vi "BlackBox Configurator.vi"() -> ()   [LabVIEW 2015]
doc: "Example VI that demonstrates all library features."
uses:
  PL BlackBox Modbus Client.lvclass
panel:
  in  "read device info":bool=TRUE
  in  "read configuration":bool=TRUE
  out "hardware interface state":T1
  in  "server configuration":T2 {"protocol" items=["RTU", "ASCII", "TCP"]}
  out "server type":u16(ring) items=["Unknown", "UART server", "Network server", "Modbus serial server", "Modbus TCP server"]
  out "hardware interface type":u16(ring) items=["Unknown", "UART", "Network interface", "Ethernet", "Wi-Fi"]
  in  "hardware interface configuration":T3 {"flow control" items=["none", "rts", "cts", "rts/cts"]; "stop bits" items=["1", "1.5", "2"]; "parity" items=["none", "even", "odd"]}
  out "server types":u16[](array[numeric])
  in  "server":u16(ring)
  out "hardware interface types":u16[](array[numeric])
  in  "hardware interface":u16(ring)
  in  "save configuration":bool
  out "uid":string
  out "firmware":string
  out "hardware":string
  in  "restart":bool
  in  "clear restarted flag":bool
  in  "device name":string
  out "PLBB":refnum<class "PL BlackBox Modbus Client.lvclass">
  in  "interface":enum32{"serial", "TCP"}(tab)
  in  "serial settings":T4={"port"="", "protocol"=enum."RTU", "address"=1, "baud rate"=115200, "data bits"=8, "parity"=2, "stop bits"=10, "flow control"=0} {"flow control" items=["None", "XON/XOFF", "RTS/CTS", "XON/XOFF & RTS/CTS", "DTR/DSR", "XON/XOFF & DTR/DSR"]; "stop bits" items=["1.0"=10, "1.5"=15, "2.0"=20]; "parity" items=["None", "Odd", "Even", "Mark", "Space"]}
  in  "TCP settings":T5={"ip address"="192.168.1.1", "port"=502, "station address"=255}
  out "error":errorcluster
  in  "stop":bool
  out "restarted":bool
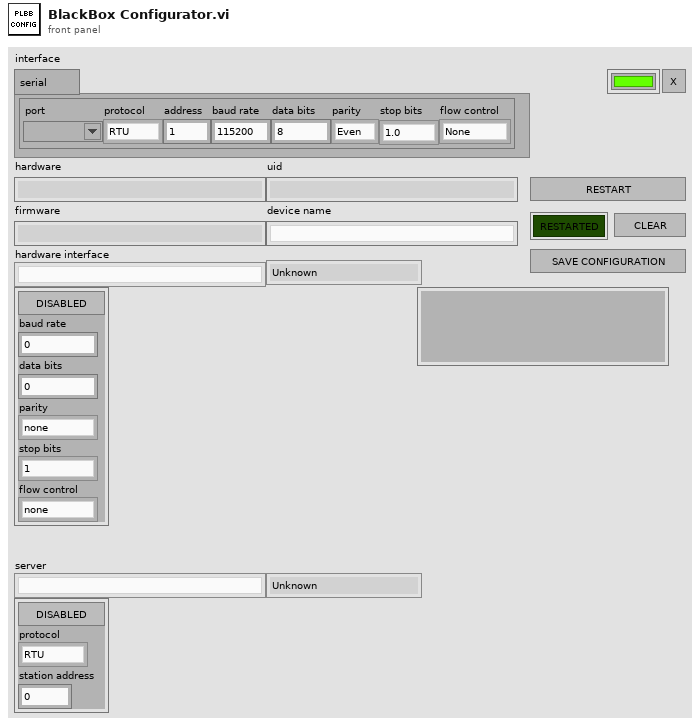
[diagram p1: front panel]
types:
  T1 = cluster{"connected":bool, "IPv6":cluster{"link-local address":string}}
  T2 = cluster{"enabled":bool, "port":u16, "max number of clients":u16, "protocol":u16, "station address":u16}
  T3 = cluster{"enabled":bool, "baud rate":u32, "data bits":u16, "parity":u16, "stop bits":u16, "flow control":u16, "IPv4":cluster{"DHCP client enabled":bool, "address":string, "netmask":string, "gateway":string}, "IPv6":cluster{"DHCP client enabled":bool, "global address":string}, "SSID":string, "password":string}
  T4 = cluster{"port":refnum<visa-resource-name>, "protocol":enum16{"RTU", "ASCII"}, "address":u8, "baud rate":u32, "data bits":u16, "parity":u16, "stop bits":u16, "flow control":u16}
  T5 = cluster{"ip address":string, "port":u16, "station address":u8}
  T6 = cluster{"connected":bool, "network interface":cluster{"IPv6":cluster{"link-local address":string}}}
  T7 = cluster{"enabled":bool, "UART":cluster{"baud rate":u32, "data bits":u16, "parity":u16, "stop bits":u16, "flow control":u16}, "network interface":cluster{"IPv4":cluster{"DHCP client enabled":bool, "address":string, "netmask":string, "gateway":string}, "IPv6":cluster{"DHCP client enabled":bool, "global address":string}, "Wi-Fi":cluster{"SSID":string, "password":string}}}
  T8 = cluster{"hardware":cluster{"name":string, "version":cluster{"major":u16, "minor":u16, "patch":u16}, "uid":string}, "firmware":cluster{"name":string, "version":cluster{"major":u16, "minor":u16, "patch":u16}}, "number of hardware interfaces":u16, "number of servers":u16}
  T9 = cluster{"DHCP client enabled":bool, "address":string, "netmask":string, "gateway":string}
  T10 = cluster{"DHCP client enabled":bool, "global address":string}
  T11 = cluster{"enabled":bool, "network server":cluster{"port":u16, "max number of clients":u16}, "Modbus server":cluster{"protocol":u16, "station address":u16}}
  T12 = cluster{"enabled":bool, "baud rate":u32, "data bits":u16, "parity":u16, "stop bits":u16, "flow control":u16}
  T13 = cluster{"enabled":bool, "IPv4":cluster{"DHCP client enabled":bool, "address":string, "netmask":string, "gateway":string}, "IPv6":cluster{"DHCP client enabled":bool, "global address":string}}
  T14 = cluster{"enabled":bool, "IPv4":cluster{"DHCP client enabled":bool, "address":string, "netmask":string, "gateway":string}, "IPv6":cluster{"DHCP client enabled":bool, "global address":string}, "SSID":string, "password":string}
  T15 = cluster{"enabled":bool, "port":u16, "max number of clients":u16}
  T16 = cluster{"enabled":bool, "protocol":u16, "station address":u16}
  T17 = cluster{"enabled":bool, "protocol":u16, "station address":u16, "port":u16, "max number of clients":u16}
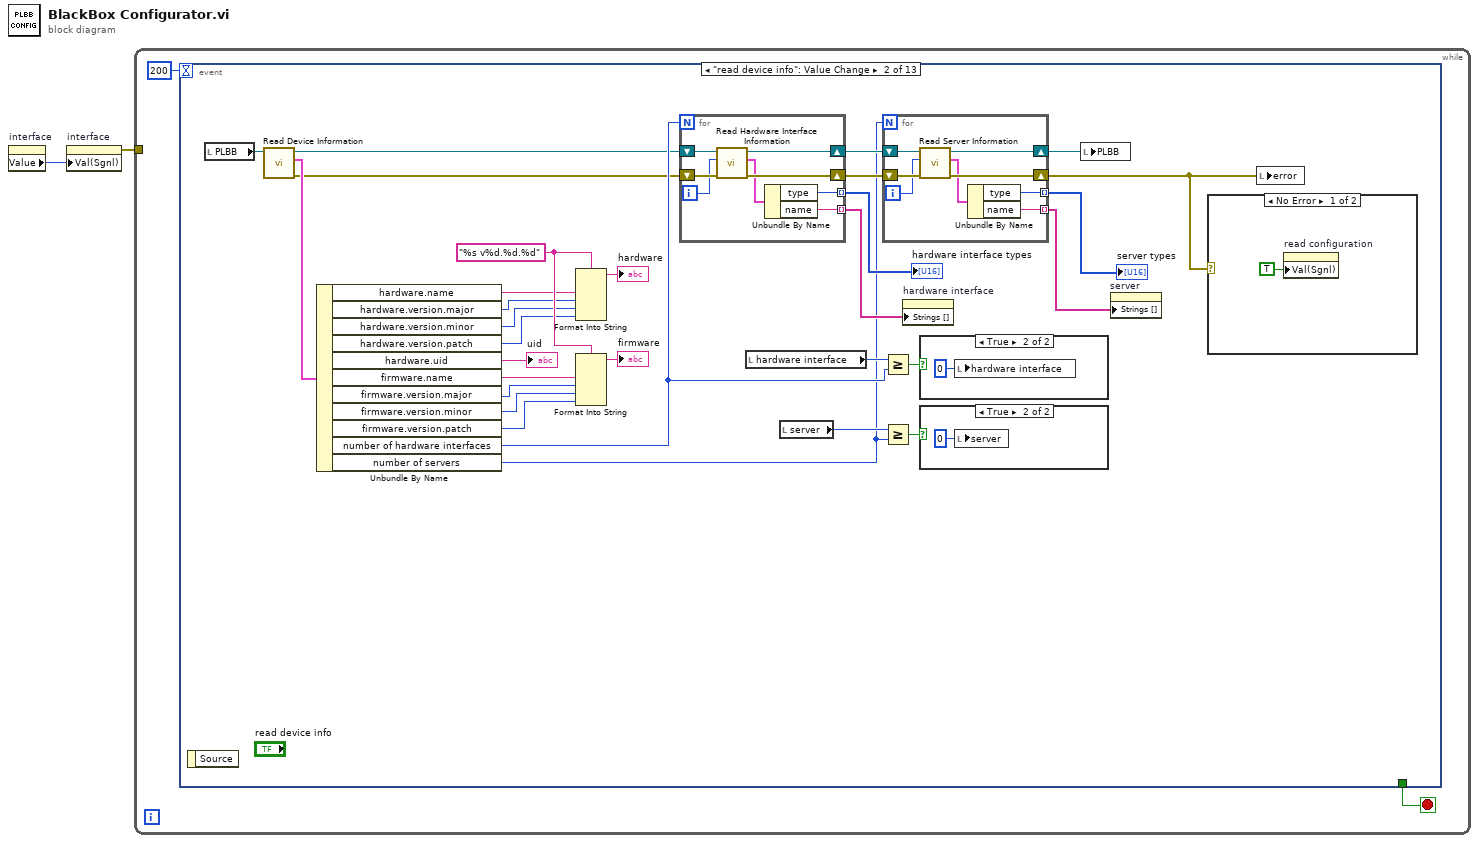
[diagram p0: block diagram]
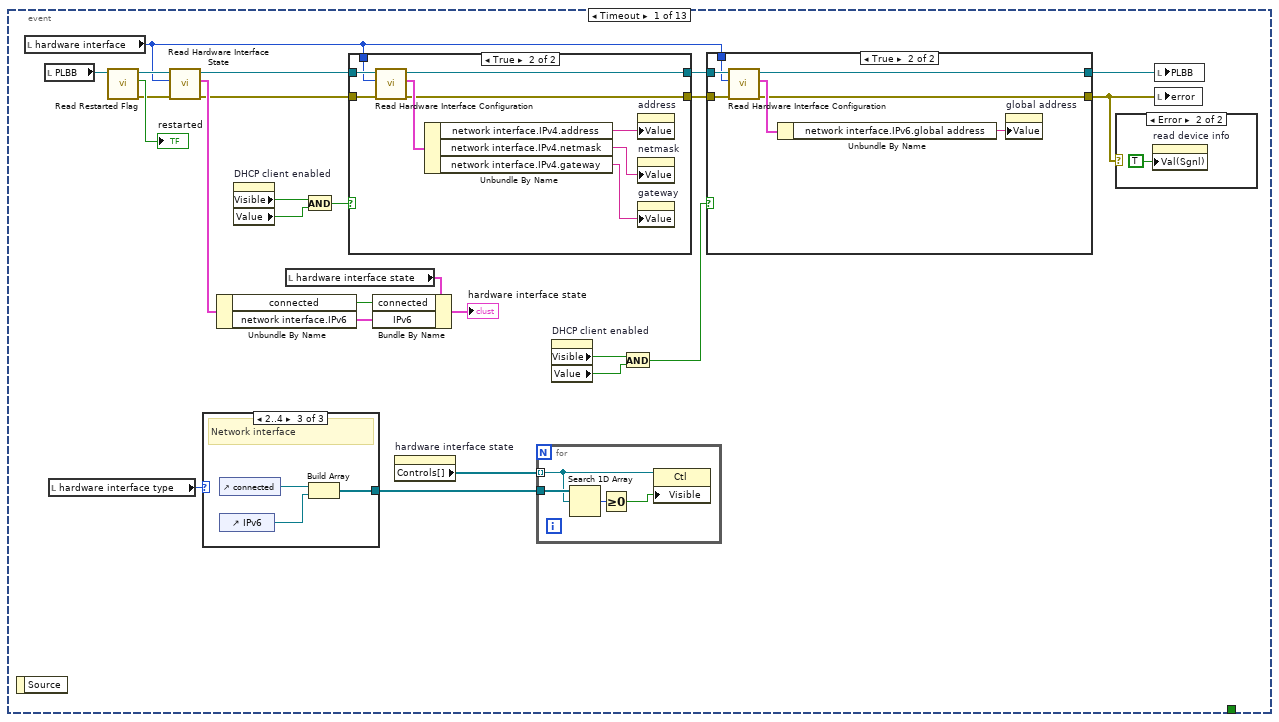
[diagram p2: hidden frame]
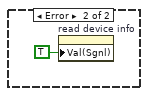
[diagram p8: hidden frame]
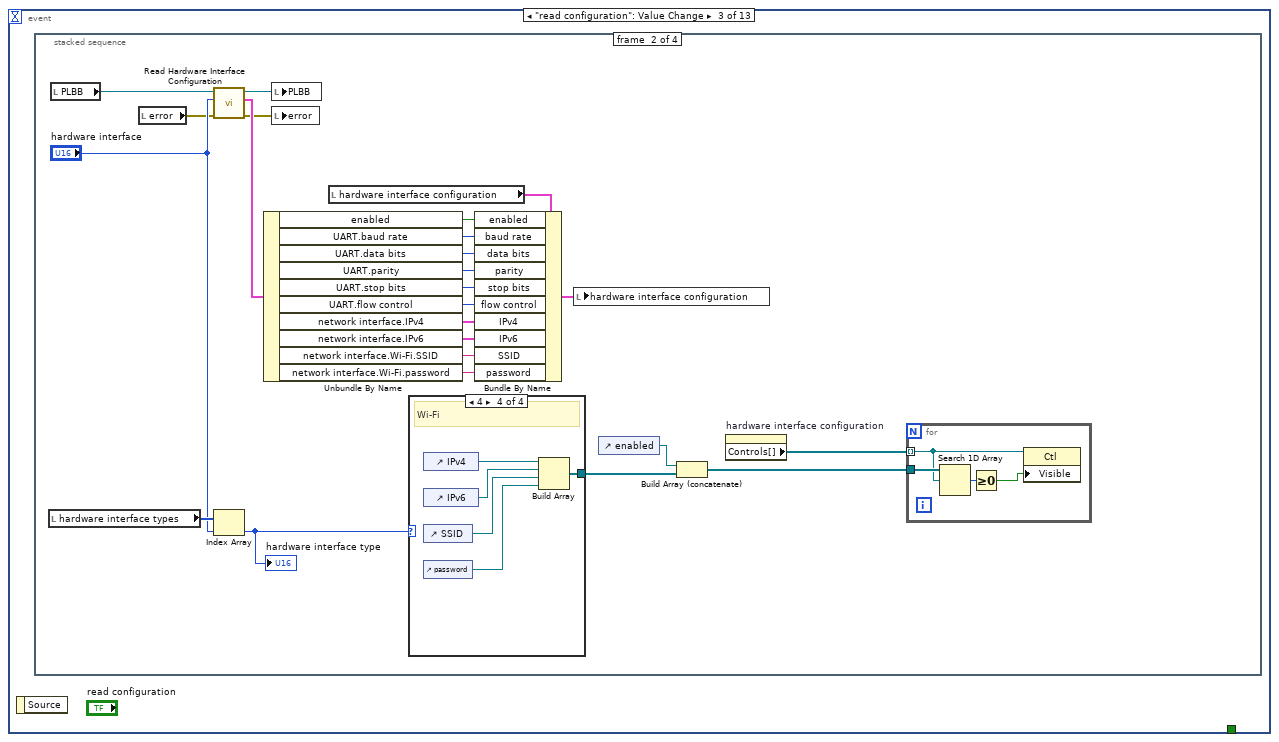
[diagram p11: hidden frame]
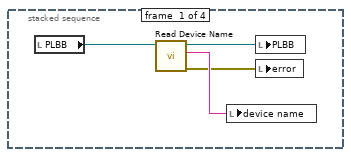
[diagram p12: hidden frame]
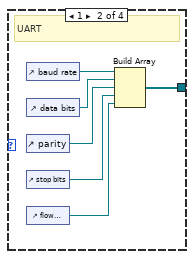
[diagram p14: hidden frame]
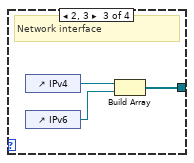
[diagram p15: hidden frame]
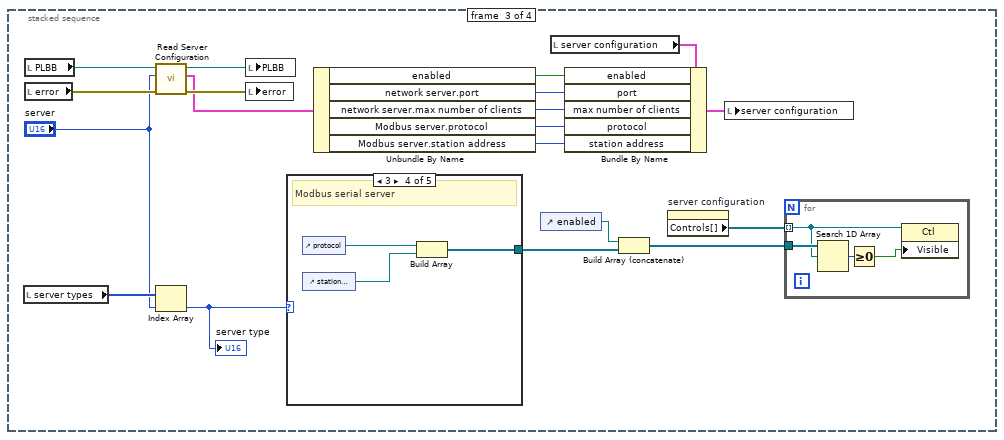
[diagram p16: hidden frame]
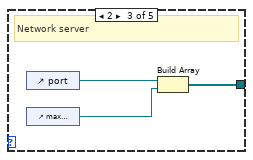
[diagram p19: hidden frame]
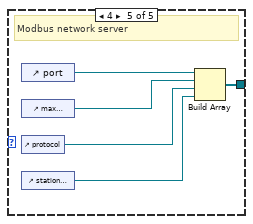
[diagram p20: hidden frame]
diagram:
  n1 = property on="interface" class="TabCtl (strict)"() -> ("Value"=w2:enum32{"serial", "TCP"})  [unwired: 2 in, 2 out]
  n2 = property on="interface" class="TabCtl (strict)"("Val(Sgnl)"=w2) -> (error out=w1:errorcluster)  [unwired: 2 in, 1 out]
  n3 = while {
    tunnel: w1 -> [_]
    stop <- w3 stop-if-true
    n4 = event shown="[1] \"read device info\": Value Change" {
      selector: _ -> [_ _ _ _ _ _ _ _ _ _ _ _ _]
      dyn-events: _ -> [_ _ _ _ _ _ _ _ _ _ _ _ _]
      timeout: 200 -> [_ _ _ _ _ _ _ _ _ _ _ _ _]
      tunnel: [_ _ _ _ _ _ _ _ _ _ _ _ TRUE ("stop")] -> w3
      event Timeout {
        n5 = event-data() -> ()  [unwired: 1 in, 1 out]
        n6 = local read "hardware interface"() -> (w13:u16)
        n7 = local read "PLBB"() -> (w24:refnum<class "PL BlackBox Modbus Client.lvclass">)
        n8 = local read "hardware interface type"() -> (w7:u16)
        n9 = call "Read Restarted Flag.vi"("PLBB in"=w24) -> ("error out"=w21:errorcluster, "restarted flag"=→"restarted":bool, "PLBB out"=w22:refnum<class "PL BlackBox Modbus Client.lvclass">)  [unwired: 8 in]
        n10 = call "Read Hardware Interface State.vi"("error in (no error)"=w21, "hardware interface index"=w13, "PLBB in"=w22) -> ("error out"=w16:errorcluster, "hardware interface state"=w28:T6, "PLBB out"=w18:refnum<class "PL BlackBox Modbus Client.lvclass">)  [unwired: 6 in]
        n11 = case shown="2..4" w7 {
          tunnel: [_ _ w36] -> w5
          frame 0, Default {
          }
          frame 1 {
            # "UART"
          }
          frame 2..4 {
            # "Network interface"
            n12 = control-ref of="connected"() -> (w34:refnum<vi>)
            n13 = control-ref of="IPv6"() -> (w35:refnum<vi>)
            n14 = Build Array(w34, w35) -> (w36:refnum<vi>[])
          }
        }
        n15 = Unbundle By Name(w28) -> ("connected"=w26:bool, "network interface.IPv6"=w25:cluster{"link-local address":string})
        n16 = property on="DHCP client enabled" class="Bool (strict)"() -> ("Visible"=w20:bool, "Value"=w19:bool)  [unwired: 2 in, 2 out]
        n17 = local read "hardware interface state"() -> (w27:T1)
        n18 = And(x=w20, y=w19) -> (x .and. y?=w17:bool)
        n19 = case shown="True" w17 {
          tunnel: w18 -> [w48 w57]
          tunnel: w16 -> [w47 w56]
          tunnel: w13 -> [_ w55]
          tunnel: [w47 w50] -> w11
          tunnel: [w48 w49] -> w12
          frame False {
          }
          frame True {
            n20 = call "Read Hardware Interface Configuration.vi"("error in (no error)"=w56, "hardware interface index"=w55, "PLBB in"=w57) -> ("error out"=w50:errorcluster, "hardware interface configuration"=w54:T7, "PLBB out"=w49:refnum<class "PL BlackBox Modbus Client.lvclass">)  [unwired: 6 in]
            n21 = Unbundle By Name(w54) -> ("network interface.IPv4.address"=w53:string, "network interface.IPv4.netmask"=w52:string, "network interface.IPv4.gateway"=w51:string)
            n22 = property on="address" class="Str"("Value"=w53) -> ()  [unwired: 2 in, 2 out]
            n23 = property on="netmask" class="Str"("Value"=w52) -> ()  [unwired: 2 in, 2 out]
            n24 = property on="gateway" class="Str"("Value"=w51) -> ()  [unwired: 2 in, 2 out]
          }
        }
        n25 = Bundle By Name(cluster=w27, "connected"=w26, "IPv6"=w25) -> (→"hardware interface state":T1)
        n26 = property on="hardware interface state" class="Clust (strict)"() -> ("Controls[]"=w6:refnum<vi>[])  [unwired: 2 in, 2 out]
        n27 = for {
          tunnel: w6 -> [w32] mode=indexing
          tunnel: w5 -> [w33]
          n28 = Search 1D Array(1D array=w33, element=w32) -> (index of element=w31:i32)  [unwired: 1 in]
          n29 = Greater Or Equal To 0?(x=w31) -> (x >= 0?=w30:bool)
          n30 = property class="Ctl"(reference=w32, "Visible"=w30) -> ()  [unwired: 1 in, 2 out]
        }
        n31 = property on="DHCP client enabled" class="Bool (strict)"() -> ("Visible"=w14:bool, "Value"=w15:bool)  [unwired: 2 in, 2 out]
        n32 = And(x=w14, y=w15) -> (x .and. y?=w9:bool)
        n33 = case shown="True" w9 {
          tunnel: w12 -> [w39 w46]
          tunnel: w11 -> [w38 w45]
          tunnel: w13 -> [_ w44]
          tunnel: [w38 w41] -> w8
          tunnel: [w39 w40] -> w10
          frame False {
          }
          frame True {
            n34 = call "Read Hardware Interface Configuration.vi"("error in (no error)"=w45, "hardware interface index"=w44, "PLBB in"=w46) -> ("error out"=w41:errorcluster, "hardware interface configuration"=w43:T7, "PLBB out"=w40:refnum<class "PL BlackBox Modbus Client.lvclass">)  [unwired: 6 in]
            n35 = Unbundle By Name(w43) -> ("network interface.IPv6.global address"=w42:string)
            n36 = property on="global address" class="Str"("Value"=w42) -> ()  [unwired: 2 in, 2 out]
          }
        }
        n37 = case shown="Error" w8 {
          frame No Error {
          }
          frame Error {
            n38 = property on="read device info" class="Bool (strict)"("Val(Sgnl)"=TRUE ("Value (Signaling)")) -> ()  [unwired: 2 in, 2 out]
          }
        }
        n39 = local write "PLBB"(w10) -> ()
        n40 = local write "error"(w8) -> ()
      }
      event "read device info": Value Change {
        w85 = "%s v%d.%d.%d" ("format string")
        n41 = event-data() -> ()  [unwired: 1 in, 1 out]
        n42 = local read "PLBB"() -> (w87:refnum<class "PL BlackBox Modbus Client.lvclass">)
        n43 = call "Read Device Information.vi"("PLBB in"=w87) -> ("error out"=w58:errorcluster, "device information"=w86:T8, "PLBB out"=w59:refnum<class "PL BlackBox Modbus Client.lvclass">)  [unwired: 8 in]
        n44 = Unbundle By Name(w86) -> ("hardware.name"=w84:string, "hardware.version.major"=w83:u16, "hardware.version.minor"=w82:u16, "hardware.version.patch"=w81:u16, "hardware.uid"=→"uid":string, "firmware.name"=w80:string, "firmware.version.major"=w79:u16, "firmware.version.minor"=w78:u16, "firmware.version.patch"=w77:u16, "number of hardware interfaces"=w64:u16, "number of servers"=w61:u16)
        n45 = Format Into String(format string=w85, w84, w83, w82, w81) -> (resulting string=→"hardware":string)  [unwired: 2 in, 1 out]
        n46 = Format Into String(format string=w85, w80, w79, w78, w77) -> (resulting string=→"firmware":string)  [unwired: 2 in, 1 out]
        n47 = for {
          N: w64 -> [_]
          shift-right: [w104] -> w69
          shift-left: w59 -> [w107]
          shift-right: [w105] -> w68
          shift-left: w58 -> [w106]
          tunnel: [w101] -> w73 mode=indexing
          tunnel: [w100] -> w72 mode=indexing
          i -> [w103]
          n48 = call "Read Hardware Interface Information.vi"("error in (no error)"=w106, "hardware interface index"=w103, "PLBB in"=w107) -> ("error out"=w105:errorcluster, "hardware interface information"=w102:cluster{"type":u16, "name":string}, "PLBB out"=w104:refnum<class "PL BlackBox Modbus Client.lvclass">)  [unwired: 6 in]
          n49 = Unbundle By Name(w102) -> ("type"=w101:u16, "name"=w100:string)
        }
        "hardware interface types" <- w73
        n50 = local read "hardware interface"() -> (w65:u16)
        n51 = local read "server"() -> (w63:u16)
        n52 = for {
          N: w61 -> [_]
          shift-right: [w96] -> w70
          shift-left: w69 -> [w99]
          shift-right: [w97] -> w60
          shift-left: w68 -> [w98]
          tunnel: [w93] -> w71 mode=indexing
          tunnel: [w92] -> w67 mode=indexing
          i -> [w95]
          n53 = call "Read Server Information.vi"("error in (no error)"=w98, "server index"=w95, "PLBB in"=w99) -> ("error out"=w97:errorcluster, "server information"=w94:cluster{"type":u16, "name":string}, "PLBB out"=w96:refnum<class "PL BlackBox Modbus Client.lvclass">)  [unwired: 6 in]
          n54 = Unbundle By Name(w94) -> ("type"=w93:u16, "name"=w92:string)
        }
        "server types" <- w71
        n55 = Greater Or Equal?(x=w65, y=w64) -> (x >= y?=w66:bool)
        n56 = Greater Or Equal?(x=w63, y=w61) -> (x >= y?=w62:bool)
        n57 = property on="hardware interface" class="Ring (strict)"("Strings []"=w72) -> ()  [unwired: 2 in, 2 out]
        n58 = case shown="True" w66 {
          frame False {
          }
          frame True {
            n59 = local write "hardware interface"(u16 0) -> ()
          }
        }
        n60 = case shown="True" w62 {
          frame False {
          }
          frame True {
            n61 = local write "server"(u16 0) -> ()
          }
        }
        n62 = local write "PLBB"(w70) -> ()
        n63 = property on="server" class="Ring (strict)"("Strings []"=w67) -> ()  [unwired: 2 in, 2 out]
        n64 = case shown="No Error" w60 {
          frame No Error {
            n65 = property on="read configuration" class="Bool (strict)"("Val(Sgnl)"=TRUE ("Value (Signaling)")) -> ()  [unwired: 2 in, 2 out]
          }
          frame Error {
            n66 = property on="read device info" class="Bool (strict)"("Val(Sgnl)"=TRUE ("Value (Signaling)")) -> ()  [unwired: 2 in, 2 out]
          }
        }
        n67 = local write "error"(w60) -> ()
      }
      event "read configuration": Value Change {
        n68 = event-data() -> ()  [unwired: 1 in, 1 out]
        n69 = stacked-sequence {
          frame #0 {
            n70 = local read "PLBB"() -> (w110:refnum<class "PL BlackBox Modbus Client.lvclass">)
            n71 = call "Read Device Name.vi"("PLBB in"=w110) -> ("error out"=w108:errorcluster, "device name"=w111:string, "PLBB out"=w109:refnum<class "PL BlackBox Modbus Client.lvclass">)  [unwired: 8 in]
            n72 = local write "device name"(w111) -> ()
            n73 = local write "PLBB"(w109) -> ()
            n74 = local write "error"(w108) -> ()
          }
          frame #1 {
            n75 = local read "hardware interface types"() -> (w134:u16[])
            n76 = local read "PLBB"() -> (w135:refnum<class "PL BlackBox Modbus Client.lvclass">)
            n77 = local read "error"() -> (w112:errorcluster)
            n78 = call "Read Hardware Interface Configuration.vi"("error in (no error)"=w112, "hardware interface index"="hardware interface", "PLBB in"=w135) -> ("error out"=w113:errorcluster, "hardware interface configuration"=w133:T7, "PLBB out"=w114:refnum<class "PL BlackBox Modbus Client.lvclass">)  [unwired: 6 in]
            n79 = Index Array(array=w134, index="hardware interface") -> (element=w122:u16)
            "hardware interface type" <- w122
            n80 = Unbundle By Name(w133) -> ("enabled"=w131:bool, "UART.baud rate"=w130:u32, "UART.data bits"=w129:u16, "UART.parity"=w128:u16, "UART.stop bits"=w127:u16, "UART.flow control"=w126:u16, "network interface.IPv4"=w125:T9, "network interface.IPv6"=w124:T10, "network interface.Wi-Fi.SSID"=w115:string, "network interface.Wi-Fi.password"=w116:string)
            n81 = local write "PLBB"(w114) -> ()
            n82 = local write "error"(w113) -> ()
            n83 = local read "hardware interface configuration"() -> (w132:T3)
            n84 = case shown="4" w122 {
              tunnel: [_ w140 w146 w149] -> w121
              frame 0, Default {
              }
              frame 1 {
                # "UART"
                n85 = control-ref of="baud rate"() -> (w141:refnum<vi>)
                n86 = control-ref of="data bits"() -> (w142:refnum<vi>)
                n87 = control-ref of="parity"() -> (w143:refnum<vi>)
                n88 = control-ref of="stop bits"() -> (w144:refnum<vi>)
                n89 = control-ref of="flow control"() -> (w145:refnum<vi>)
                n90 = Build Array(w141, w142, w143, w144, w145) -> (w140:refnum<vi>[])
              }
              frame 2, 3 {
                # "Network interface"
                n91 = control-ref of="IPv4"() -> (w147:refnum<vi>)
                n92 = control-ref of="IPv6"() -> (w148:refnum<vi>)
                n93 = Build Array(w147, w148) -> (w146:refnum<vi>[])
              }
              frame 4 {
                # "Wi-Fi"
                n94 = control-ref of="IPv4"() -> (w150:refnum<vi>)
                n95 = control-ref of="IPv6"() -> (w151:refnum<vi>)
                n96 = control-ref of="SSID"() -> (w152:refnum<vi>)
                n97 = control-ref of="password"() -> (w153:refnum<vi>)
                n98 = Build Array(w150, w151, w152, w153) -> (w149:refnum<vi>[])
              }
            }
            n99 = Bundle By Name(cluster=w132, "enabled"=w131, "baud rate"=w130, "data bits"=w129, "parity"=w128, "stop bits"=w127, "flow control"=w126, "IPv4"=w125, "IPv6"=w124, "SSID"=w115, "password"=w116) -> (w123:T3)
            n100 = local write "hardware interface configuration"(w123) -> ()
            n101 = control-ref of="enabled"() -> (w120:refnum<vi>)
            n102 = Build Array (concatenate)(w120, w121) -> (w118:refnum<vi>[])
            n103 = property on="hardware interface configuration" class="Clust (strict)"() -> ("Controls[]"=w119:refnum<vi>[])  [unwired: 2 in, 2 out]
            n104 = for {
              tunnel: w119 -> [w138] mode=indexing
              tunnel: w118 -> [w139]
              n105 = Search 1D Array(1D array=w139, element=w138) -> (index of element=w137:i32)  [unwired: 1 in]
              n106 = Greater Or Equal To 0?(x=w137) -> (x >= 0?=w136:bool)
              n107 = property class="Ctl"(reference=w138, "Visible"=w136) -> ()  [unwired: 1 in, 2 out]
            }
          }
          frame #2 {
            n108 = local read "server types"() -> (w168:u16[])
            n109 = local read "PLBB"() -> (w172:refnum<class "PL BlackBox Modbus Client.lvclass">)
            n110 = local read "error"() -> (w171:errorcluster)
            n111 = call "Read Server Configuration.vi"("error in (no error)"=w171, "server index"="server", "PLBB in"=w172) -> ("error out"=w169:errorcluster, "server configuration"=w167:T11, "PLBB out"=w170:refnum<class "PL BlackBox Modbus Client.lvclass">)  [unwired: 6 in]
            n112 = Index Array(array=w168, index="server") -> (element=w154:u16)
            "server type" <- w154
            n113 = local write "PLBB"(w170) -> ()
            n114 = local write "error"(w169) -> ()
            n115 = case shown="3" w154 {
              tunnel: [_ _ w177 w180 w183] -> w159
              frame 0, Default {
              }
              frame 1 {
                # "UART server"
              }
              frame 2 {
                # "Network server"
                n116 = control-ref of="port"() -> (w178:refnum<vi>)
                n117 = control-ref of="max number of clients"() -> (w179:refnum<vi>)
                n118 = Build Array(w178, w179) -> (w177:refnum<vi>[])
              }
              frame 3 {
                # "Modbus serial server"
                n119 = control-ref of="protocol"() -> (w181:refnum<vi>)
                n120 = control-ref of="station address"() -> (w182:refnum<vi>)
                n121 = Build Array(w181, w182) -> (w180:refnum<vi>[])
              }
              frame 4 {
                # "Modbus network server"
                n122 = control-ref of="port"() -> (w184:refnum<vi>)
                n123 = control-ref of="max number of clients"() -> (w185:refnum<vi>)
                n124 = control-ref of="protocol"() -> (w186:refnum<vi>)
                n125 = control-ref of="station address"() -> (w187:refnum<vi>)
                n126 = Build Array(w184, w185, w186, w187) -> (w183:refnum<vi>[])
              }
            }
            n127 = Unbundle By Name(w167) -> ("enabled"=w165:bool, "network server.port"=w164:u16, "network server.max number of clients"=w163:u16, "Modbus server.protocol"=w162:u16, "Modbus server.station address"=w161:u16)
            n128 = control-ref of="enabled"() -> (w158:refnum<vi>)
            n129 = local read "server configuration"() -> (w166:T2)
            n130 = Bundle By Name(cluster=w166, "enabled"=w165, "port"=w164, "max number of clients"=w163, "protocol"=w162, "station address"=w161) -> (w160:T2)
            n131 = Build Array (concatenate)(w158, w159) -> (w156:refnum<vi>[])
            n132 = property on="server configuration" class="Clust (strict)"() -> ("Controls[]"=w157:refnum<vi>[])  [unwired: 2 in, 2 out]
            n133 = local write "server configuration"(w160) -> ()
            n134 = for {
              tunnel: w157 -> [w175] mode=indexing
              tunnel: w156 -> [w176]
              n135 = Search 1D Array(1D array=w176, element=w175) -> (index of element=w174:i32)  [unwired: 1 in]
              n136 = Greater Or Equal To 0?(x=w174) -> (x >= 0?=w173:bool)
              n137 = property class="Ctl"(reference=w175, "Visible"=w173) -> ()  [unwired: 1 in, 2 out]
            }
          }
          frame #3 {
            n138 = local read "error"() -> (w188:errorcluster)
            n139 = case shown="Error" w188 {
              frame No Error {
              }
              frame Error {
                n140 = property on="read device info" class="Bool (strict)"("Val(Sgnl)"=TRUE ("Value (Signaling)")) -> ()  [unwired: 2 in, 2 out]
              }
            }
          }
        }
      }
      event "restart": Value Change {
        n141 = event-data() -> ()  [unwired: 1 in, 1 out]
        n142 = local read "PLBB"() -> (w190:refnum<class "PL BlackBox Modbus Client.lvclass">)
        n143 = call "Restart.vi"("PLBB in"=w190) -> ("error out"=w192:errorcluster, "PLBB out"=w191:refnum<class "PL BlackBox Modbus Client.lvclass">)  [unwired: 9 in]
        n144 = local write "PLBB"(w191) -> ()
        n145 = local write "error"(w192) -> ()
      }
      event "clear restarted flag": Value Change {
        n146 = event-data() -> ()  [unwired: 1 in, 1 out]
        n147 = local read "PLBB"() -> (w193:refnum<class "PL BlackBox Modbus Client.lvclass">)
        n148 = call "Clear Restarted Flag.vi"("PLBB in"=w193) -> ("error out"=w195:errorcluster, "PLBB out"=w194:refnum<class "PL BlackBox Modbus Client.lvclass">)  [unwired: 9 in]
        n149 = local write "PLBB"(w194) -> ()
        n150 = local write "error"(w195) -> ()
      }
      event "save configuration": Value Change {
        n151 = event-data() -> ()  [unwired: 1 in, 1 out]
        n152 = local read "PLBB"() -> (w196:refnum<class "PL BlackBox Modbus Client.lvclass">)
        n153 = call "Save Configuration.vi"("PLBB in"=w196) -> ("error out"=w198:errorcluster, "PLBB out"=w197:refnum<class "PL BlackBox Modbus Client.lvclass">)  [unwired: 9 in]
        n154 = local write "PLBB"(w197) -> ()
        n155 = local write "error"(w198) -> ()
      }
      event "device name": Value Change {
        n156 = event-data() -> ()  [unwired: 1 in, 1 out]
        n157 = local read "PLBB"() -> (w201:refnum<class "PL BlackBox Modbus Client.lvclass">)
        n158 = call "Write Device Name.vi"("device name"="device name", "PLBB in"=w201) -> ("error out"=w203:errorcluster, "PLBB out"=w202:refnum<class "PL BlackBox Modbus Client.lvclass">)  [unwired: 8 in]
        n159 = local write "PLBB"(w202) -> ()
        n160 = local write "error"(w203) -> ()
        n161 = property on="read configuration" class="Bool (strict)"("Val(Sgnl)"=TRUE ("Value (Signaling)")) -> ()  [unwired: 2 in, 2 out]
      }
      event "hardware interface", "server": Value Change {
        n162 = event-data() -> ()  [unwired: 1 in, 6 out]
        n163 = property on="read configuration" class="Bool (strict)"("Val(Sgnl)"=TRUE ("Value (Signaling)")) -> ()  [unwired: 2 in, 2 out]
      }
      event "hardware interface configuration": Value Change {
        n164 = event-data() -> ("NewVal"=w210:T3)  [unwired: 1 in]
        n165 = local read "hardware interface type"() -> (w211:u16)
        n166 = local read "hardware interface"() -> (w206:u16)
        n167 = local read "PLBB"() -> (w209:refnum<class "PL BlackBox Modbus Client.lvclass">)
        n168 = case shown="4" w211 {
          tunnel: w210 -> [w214 w226 w235 w244 w255]
          tunnel: w209 -> [w218 w230 w239 w248 w259]
          tunnel: [w217 w229 w238 w247 w258] -> w208
          tunnel: [w216 w228 w237 w246 w257] -> w207
          tunnel: w206 -> [w215 w227 w236 w245 w256]
          frame 0, Default {
            n169 = Unbundle By Name(w214) -> ("enabled"=w213:bool)
            n170 = Bundle("enabled"=w213) -> (w212:cluster{"enabled":bool})  [unwired: 1 in]
            n171 = call "Configure Hardware Interface.vi"("hardware interface configuration"=w212, "hardware interface index"=w215, "PLBB in"=w218) -> ("error out"=w216:errorcluster, "PLBB out"=w217:refnum<class "PL BlackBox Modbus Client.lvclass">)  [unwired: 7 in]
          }
          frame 1 {
            # "UART"
            n172 = Unbundle By Name(w226) -> ("enabled"=w225:bool, "baud rate"=w224:u32, "data bits"=w223:u16, "parity"=w222:u16, "stop bits"=w221:u16, "flow control"=w220:u16)
            n173 = Bundle("enabled"=w225, "baud rate"=w224, "data bits"=w223, "parity"=w222, "stop bits"=w221, "flow control"=w220) -> (w219:T12)  [unwired: 1 in]
            n174 = call "Configure UART.vi"("UART configuration"=w219, "hardware interface index"=w227, "PLBB in"=w230) -> ("error out"=w228:errorcluster, "PLBB out"=w229:refnum<class "PL BlackBox Modbus Client.lvclass">)  [unwired: 7 in]
          }
          frame 2 {
            # "Network interface"
            n175 = Unbundle By Name(w235) -> ("enabled"=w234:bool, "IPv4"=w233:T9, "IPv6"=w232:T10)
            n176 = Bundle("enabled"=w234, "IPv4"=w233, "IPv6"=w232) -> (w231:T13)  [unwired: 1 in]
            n177 = call "Configure Network Interface.vi"("network interface configuration"=w231, "hardware interface index"=w236, "PLBB in"=w239) -> ("error out"=w237:errorcluster, "PLBB out"=w238:refnum<class "PL BlackBox Modbus Client.lvclass">)  [unwired: 7 in]
          }
          frame 3 {
            # "Ethernet"
            n178 = Unbundle By Name(w244) -> ("enabled"=w243:bool, "IPv4"=w242:T9, "IPv6"=w241:T10)
            n179 = Bundle("enabled"=w243, "IPv4"=w242, "IPv6"=w241) -> (w240:T13)  [unwired: 1 in]
            n180 = call "Configure Ethernet.vi"("Ethernet configuration"=w240, "hardware interface index"=w245, "PLBB in"=w248) -> ("error out"=w246:errorcluster, "PLBB out"=w247:refnum<class "PL BlackBox Modbus Client.lvclass">)  [unwired: 7 in]
          }
          frame 4 {
            # "Wi-Fi"
            n181 = Unbundle By Name(w255) -> ("enabled"=w254:bool, "IPv4"=w253:T9, "IPv6"=w252:T10, "SSID"=w250:string, "password"=w249:string)
            n182 = Bundle("enabled"=w254, "IPv4"=w253, "IPv6"=w252, "SSID"=w250, "password"=w249) -> (w251:T14)  [unwired: 1 in]
            n183 = call "Configure Wi-Fi.vi"("Wi-Fi configuration"=w251, "hardware interface index"=w256, "PLBB in"=w259) -> ("error out"=w257:errorcluster, "PLBB out"=w258:refnum<class "PL BlackBox Modbus Client.lvclass">)  [unwired: 7 in]
          }
        }
        n184 = local write "PLBB"(w208) -> ()
        n185 = local write "error"(w207) -> ()
        n186 = property on="read configuration" class="Bool (strict)"("Val(Sgnl)"=TRUE ("Value (Signaling)")) -> ()  [unwired: 2 in, 2 out]
      }
      event "server configuration": Value Change {
        n187 = event-data() -> ("NewVal"=w265:T2)  [unwired: 1 in]
        n188 = local read "server type"() -> (w266:u16)
        n189 = local read "PLBB"() -> (w264:refnum<class "PL BlackBox Modbus Client.lvclass">)
        n190 = local read "server"() -> (w261:u16)
        n191 = case shown="0, Default" w266 {
          tunnel: w265 -> [w269 w276 w285 w294 w305]
          tunnel: w264 -> [w273 w280 w289 w298 w309]
          tunnel: [w272 w279 w288 w297 w308] -> w263
          tunnel: [w271 w278 w287 w296 w307] -> w262
          tunnel: w261 -> [w270 w277 w286 w295 w306]
          frame 0, Default {
            n192 = Unbundle By Name(w269) -> ("enabled"=w268:bool)
            n193 = Bundle("enabled"=w268) -> (w267:cluster{"enabled":bool})  [unwired: 1 in]
            n194 = call "Configure Server.vi"("server configuration"=w267, "server index"=w270, "PLBB in"=w273) -> ("error out"=w271:errorcluster, "PLBB out"=w272:refnum<class "PL BlackBox Modbus Client.lvclass">)  [unwired: 7 in]
          }
          frame 1 {
            # "UART server"
            n195 = Unbundle By Name(w276) -> ("enabled"=w275:bool)
            n196 = Bundle("enabled"=w275) -> (w274:cluster{"enabled":bool})  [unwired: 1 in]
            n197 = call "Configure UART Server.vi"("UART server configuration"=w274, "server index"=w277, "PLBB in"=w280) -> ("error out"=w278:errorcluster, "PLBB out"=w279:refnum<class "PL BlackBox Modbus Client.lvclass">)  [unwired: 7 in]
          }
          frame 2 {
            # "Network server"
            n198 = Unbundle By Name(w285) -> ("enabled"=w284:bool, "port"=w283:u16, "max number of clients"=w282:u16)
            n199 = Bundle("enabled"=w284, "port"=w283, "max number of clients"=w282) -> (w281:T15)  [unwired: 1 in]
            n200 = call "Configure Network Server.vi"("network server configuration"=w281, "server index"=w286, "PLBB in"=w289) -> ("error out"=w287:errorcluster, "PLBB out"=w288:refnum<class "PL BlackBox Modbus Client.lvclass">)  [unwired: 7 in]
          }
          frame 3 {
            # "Modbus serial server"
            n201 = Unbundle By Name(w294) -> ("enabled"=w293:bool, "protocol"=w292:u16, "station address"=w291:u16)
            n202 = Bundle("enabled"=w293, "protocol"=w292, "station address"=w291) -> (w290:T16)  [unwired: 1 in]
            n203 = call "Configure Modbus Serial Server.vi"("Modbus serial server configuration"=w290, "server index"=w295, "PLBB in"=w298) -> ("error out"=w296:errorcluster, "PLBB out"=w297:refnum<class "PL BlackBox Modbus Client.lvclass">)  [unwired: 7 in]
          }
          frame 4 {
            # "Modbus TCP server"
            n204 = Unbundle By Name(w305) -> ("enabled"=w304:bool, "protocol"=w303:u16, "station address"=w302:u16, "port"=w301:u16, "max number of clients"=w300:u16)
            n205 = Bundle("enabled"=w304, "protocol"=w303, "station address"=w302, "port"=w301, "max number of clients"=w300) -> (w299:T17)  [unwired: 1 in]
            n206 = call "Configure Modbus TCP Server.vi"("Modbus TCP server configuration"=w299, "server index"=w306, "PLBB in"=w309) -> ("error out"=w307:errorcluster, "PLBB out"=w308:refnum<class "PL BlackBox Modbus Client.lvclass">)  [unwired: 7 in]
          }
        }
        n207 = local write "PLBB"(w263) -> ()
        n208 = local write "error"(w262) -> ()
        n209 = property on="read configuration" class="Bool (strict)"("Val(Sgnl)"=TRUE ("Value (Signaling)")) -> ()  [unwired: 2 in, 2 out]
      }
      event "interface", "serial settings", "TCP settings": Value Change {
        n210 = event-data() -> ()  [unwired: 1 in, 6 out]
        n211 = local read "PLBB"() -> (w315:refnum<class "PL BlackBox Modbus Client.lvclass">)
        n212 = call-dynamic "Close.vi"("PLBB in"=w315) -> ("error out"=w316:errorcluster)  [unwired: 10 in]
        n213 = call <vilib>:"Clear Errors.vi"("error in (no error)"=w316) -> ("error out"=w313:errorcluster)  [unwired: 5 in, 1 out]
        n214 = case shown="\"serial\", Default" "interface" {
          tunnel: [w327 w333] -> w312
          tunnel: [w326 w332] -> w311
          tunnel: w313 -> [_ _]
          frame "serial", Default {
            n215 = Unbundle By Name("serial settings") -> ("address"=w318:u8, "protocol"=w319:enum16{"RTU", "ASCII"}, "port"=w321:refnum<visa-resource-name>, "baud rate"=w320:u32, "data bits"=w322:u16, "parity"=w323:u16, "stop bits"=w324:u16, "flow control"=w325:u16)
            n216 = call "Initialize BlackBox Modbus Client Serial.vi"("protocol (RTU)"=w319, "station address (1)"=w318, "port"=w321, "baud rate (115200)"=w320, "data bits (8)"=w322, "parity (even)"=w323, "stop bits (1.0)"=w324, "flow control (none)"=w325) -> ("PLBB out"=w327:refnum<class "PL BlackBox Modbus Client.lvclass">, "error out"=w326:errorcluster)  [unwired: 6 in]
          }
          frame "TCP" {
            n217 = Unbundle By Name("TCP settings") -> ("ip address"=w330:string, "port"=w329:u16, "station address"=w328:u8)
            n218 = call "Initialize BlackBox Modbus Client TCP.vi"("station address (255)"=w328, "port (502)"=w329, "ip address"=w330) -> ("error out"=w332:errorcluster, "PLBB out"=w333:refnum<class "PL BlackBox Modbus Client.lvclass">)  [unwired: 7 in]
          }
        }
        "error" <- w311
        "PLBB" <- w312
        n219 = property on="read device info" class="Bool (strict)"("Val(Sgnl)"=TRUE ("Value (Signaling)")) -> ()  [unwired: 2 in, 2 out]
      }
      event "error": Mouse Up {
        n220 = event-data() -> ()  [unwired: 1 in, 1 out]
        n221 = local read "error"() -> (w334:errorcluster)
        n222 = call <vilib>:"Simple Error Handler.vi"("error in (no error)"=w334) -> ()  [unwired: 4 in, 5 out]
      }
      event "stop": Value Change {
        n223 = event-data() -> ()  [unwired: 1 in, 1 out]
        n224 = local read "PLBB"() -> (w336:refnum<class "PL BlackBox Modbus Client.lvclass">)
        n225 = call-dynamic "Close.vi"("PLBB in"=w336) -> ("error out"=w335:errorcluster)  [unwired: 10 in]
        n226 = call <vilib>:"Clear Errors.vi"("error in (no error)"=w335) -> ()  [unwired: 5 in, 2 out]
      }
    }
  }
